vi "Capture_and_read.vi"() -> ()   [LabVIEW 2018]
panel:
  in  "FIBER":u32=1 min=1 max=20 step=1
  out "SATURATION":u32
  out "INTENSITY":u32
  out "HUE":dbl
  in  "VISA resource name":refnum<visa-resource-name>="ASRL34::INSTR"
  out "OUTPUT":string
  # "NOTE: remember plug-in the LED Analyser\ncable before run this VI and to select the\nVISA resource name (port)"
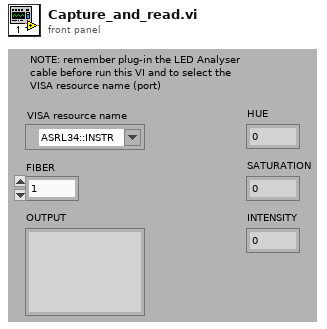
[diagram p1: front panel]
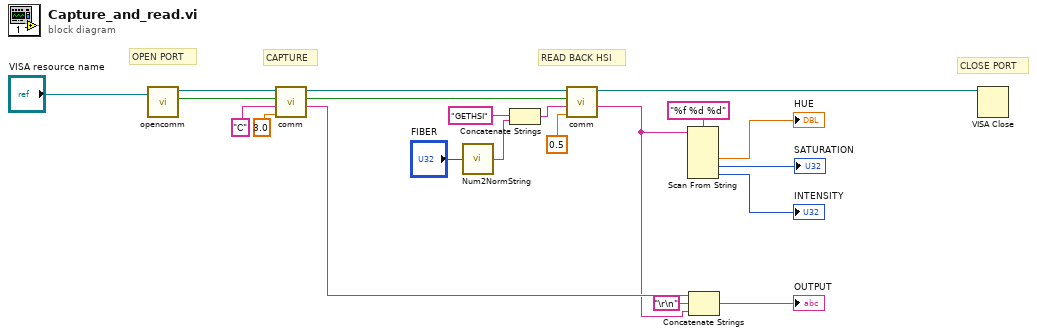
[diagram p0: block diagram]
diagram:
  # "CLOSE PORT"
  # "READ BACK HSI"
  # "CAPTURE"
  # "OPEN PORT"
  n1 = call "opencomm.vi"("VISA resource name"="VISA resource name") -> ("duplicate VISA resource name"=w19:refnum<visa-resource-name>, "Error"=w18:bool)  [unwired: 3 in]
  n2 = call "comm.vi"("Timeout (s)"=3.0, "Command"="C", "Error"=w18, "VISA resource name"=w19) -> ("Response"=w8:string, "Error"=w16:bool, "dup VISA resource name"=w17:refnum<visa-resource-name>)  [unwired: 2 in, 1 out]
  n3 = call "Num2NormString.vi"("Number"="FIBER") -> ("Normalized String Number"=w13:string)
  n4 = Concatenate Strings("GETHSI" ("Command"), w13) -> (w12:string)
  n5 = call "comm.vi"("Timeout (s)"=0.5, "Command"=w12, "Error"=w16, "VISA resource name"=w17) -> ("Response"=w5:string, "dup VISA resource name"=w10:refnum<visa-resource-name>)  [unwired: 2 in, 2 out]
  n6 = Scan From String(format string="%f %d %d", input string=w5) -> (output 1=→"HUE":dbl, output 2=→"SATURATION":u32, output 3=→"INTENSITY":u32)  [unwired: 5 in, 3 out]
  n7 = Concatenate Strings(w8, "\r\n", w5) -> (→"OUTPUT":string)
  n8 = VISA Close(VISA resource name=w10) -> ()  [unwired: 1 in, 1 out]
